vi "Hora_Solar.vi"(0 "Grados":i32, 1 "Min":i32, 2 "Seg":i32, 8 "Hora Oficial":i32, 9 "Min Oficial":i32, 10 "Seg Oficial":i32, 11 "Día del año (n)":dbl) -> (3 "Eq. Tiempo":dbl, 4 "Min Solar":i32, 5 "Hora Solar":dbl, 6 "Hr Solar":i32, 7 "Seg Solar":i32)   [LabVIEW 2020]
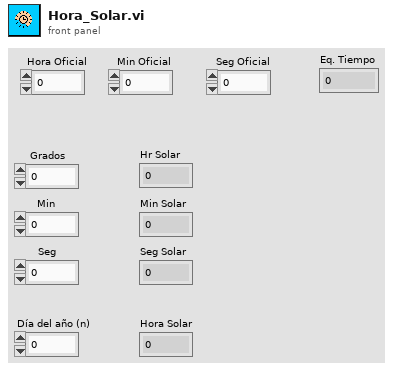
[diagram p1: front panel]
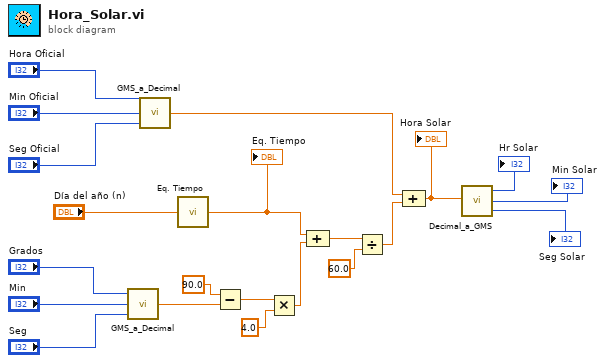
[diagram p0: block diagram]
diagram:
  n1 = call "GMS_a_Decimal.vi"("Segundos"="Seg", "Minutos"="Min", "Grados"="Grados") -> ("Decimal"=w15:dbl)
  n2 = call "GMS_a_Decimal.vi"("Segundos"="Seg Oficial", "Minutos"="Min Oficial", "Grados"="Hora Oficial") -> ("Decimal"=w7:dbl)
  n3 = call "Eq. Tiempo.vi"("Día del año (n)"="Día del año (n)") -> ("Eq. Tiempo"=w1:dbl)
  "Eq. Tiempo" <- w1
  n4 = Subtract(x=90.0, y=w15) -> (x-y=w13:dbl)
  n5 = Multiply(x=w13, y=4.0) -> (x*y=w11:dbl)
  n6 = Compound Arithmetic op=ADD(w1, w11) -> (w10:dbl)
  n7 = Divide(x=w10, y=60.0) -> (x/y=w8:dbl)
  n8 = Compound Arithmetic op=ADD(w7, w8) -> (w6:dbl)
  "Hora Solar" <- w6
  n9 = call "Decimal_a_GMS.vi"("Decimal"=w6) -> ("Grados"=→"Hr Solar":i32, "Minutos"=→"Min Solar":i32, "Segundos"=→"Seg Solar":i32)
